vi "myRIO_BRig_Host_formatData_getPaths.vi"(0 "input_storagePath":string="C:\\BehaviorRig\\Data\\2016_03_02__Exp1_TM2_run3") -> (13 "output_dataTrial":string, 14 "output_dataBlock":string, 15 "output_dataCurrent":string, 16 "output_dataExp":string, 17 "output_dataLC":string, 18 "output_dataLick":string, 19 "output_dataMTrig":string)   [LabVIEW 2014]
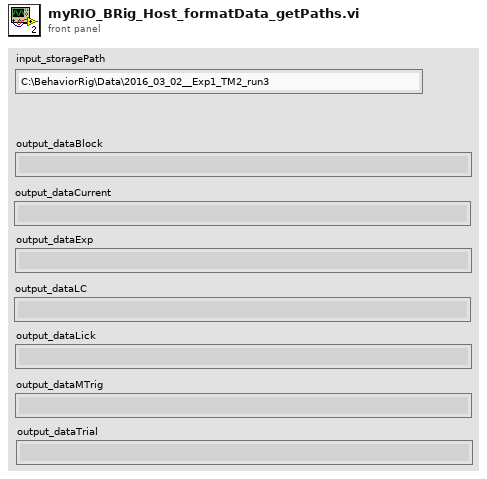
[diagram p1: front panel]
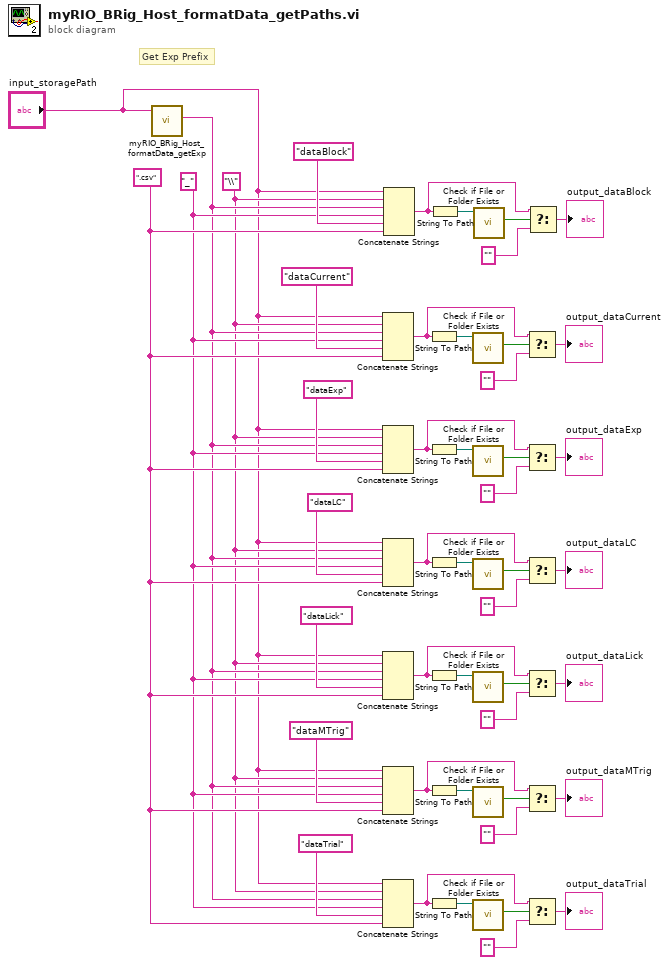
[diagram p0: block diagram]
diagram:
  w5 = ".csv" ("string")
  w4 = "_" ("string")
  w2 = "\\" ("string")
  # "Get Exp Prefix"
  n1 = call "myRIO_BRig_Host_formatData_getExp.vi"("input_folderPath"="input_storagePath") -> ("output_ExpPrefix"=w3:string)  [unwired: 10 in]
  n2 = Concatenate Strings("input_storagePath", w2, w3, w4, "dataCurrent" ("string"), w5) -> (w38:string)
  n3 = Concatenate Strings("input_storagePath", w2, w3, w4, "dataExp" ("string"), w5) -> (w32:string)
  n4 = Concatenate Strings("input_storagePath", w2, w3, w4, "dataLC" ("string"), w5) -> (w26:string)
  n5 = Concatenate Strings("input_storagePath", w2, w3, w4, "dataLick" ("string"), w5) -> (w20:string)
  n6 = Concatenate Strings("input_storagePath", w2, w3, w4, "dataMTrig" ("string"), w5) -> (w14:string)
  n7 = Concatenate Strings("input_storagePath", w2, w3, w4, "dataTrial" ("string"), w5) -> (w8:string)
  n8 = Concatenate Strings("input_storagePath", w2, w3, w4, "dataBlock" ("string"), w5) -> (w44:string)
  n9 = String To Path(string=w38) -> (path=w40:path)
  n10 = String To Path(string=w32) -> (path=w34:path)
  n11 = String To Path(string=w26) -> (path=w28:path)
  n12 = String To Path(string=w20) -> (path=w22:path)
  n13 = String To Path(string=w14) -> (path=w16:path)
  n14 = String To Path(string=w8) -> (path=w10:path)
  n15 = String To Path(string=w44) -> (path=w46:path)
  n16 = call <vilib>:"Check if File or Folder Exists.vi"("path"=w40) -> ("file or folder exists?"=w39:bool)  [unwired: 8 in, 2 out]
  n17 = call <vilib>:"Check if File or Folder Exists.vi"("path"=w34) -> ("file or folder exists?"=w33:bool)  [unwired: 8 in, 2 out]
  n18 = call <vilib>:"Check if File or Folder Exists.vi"("path"=w28) -> ("file or folder exists?"=w27:bool)  [unwired: 8 in, 2 out]
  n19 = call <vilib>:"Check if File or Folder Exists.vi"("path"=w22) -> ("file or folder exists?"=w21:bool)  [unwired: 8 in, 2 out]
  n20 = call <vilib>:"Check if File or Folder Exists.vi"("path"=w16) -> ("file or folder exists?"=w15:bool)  [unwired: 8 in, 2 out]
  n21 = call <vilib>:"Check if File or Folder Exists.vi"("path"=w10) -> ("file or folder exists?"=w9:bool)  [unwired: 8 in, 2 out]
  n22 = call <vilib>:"Check if File or Folder Exists.vi"("path"=w46) -> ("file or folder exists?"=w45:bool)  [unwired: 8 in, 2 out]
  n23 = Select(t=w38, s=w39, f="") -> (s? t:f=→"output_dataCurrent":string)
  n24 = Select(t=w32, s=w33, f="") -> (s? t:f=→"output_dataExp":string)
  n25 = Select(t=w26, s=w27, f="") -> (s? t:f=→"output_dataLC":string)
  n26 = Select(t=w20, s=w21, f="") -> (s? t:f=→"output_dataLick":string)
  n27 = Select(t=w14, s=w15, f="") -> (s? t:f=→"output_dataMTrig":string)
  n28 = Select(t=w8, s=w9, f="") -> (s? t:f=→"output_dataTrial":string)
  n29 = Select(t=w44, s=w45, f="") -> (s? t:f=→"output_dataBlock":string)
